vi "Get Grouped Channel Settings.vi"(9 "Type":T2(ring), 10 "Group Name":string, 11 "Group Settings":T3(array[cluster])) -> (1 "found?":bool, 2 "Channel Settings":T1(array[cluster]), 3 "Name based Group Settings":T3(array[cluster]))   [LabVIEW 2026, in "Template.lvlib" / "Template.lvclass"]
uses:
  Template.lvclass
  Template.lvclass/Template.ctl
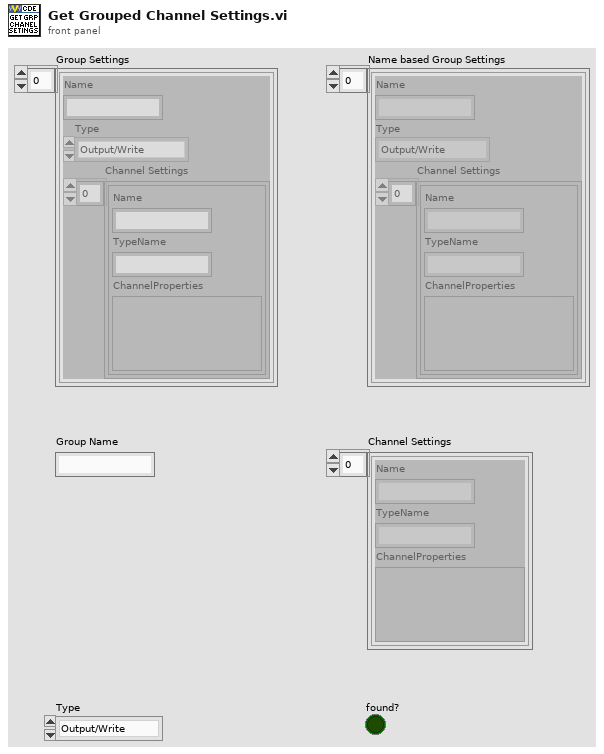
[diagram p1: front panel]
types:
  T1 = cluster{"Name":string, "TypeName":string, "ChannelProperties":variant}[]
  T2 = enum16{"Output/Write", "Input/Read", "Input/ReadWrite"}
  T3 = cluster{"Name":string, "Type":enum16{"Output/Write", "Input/Read", "Input/ReadWrite"}, "Channel Settings":cluster{"Name":string, "TypeName":string, "ChannelProperties":variant}[]}[]
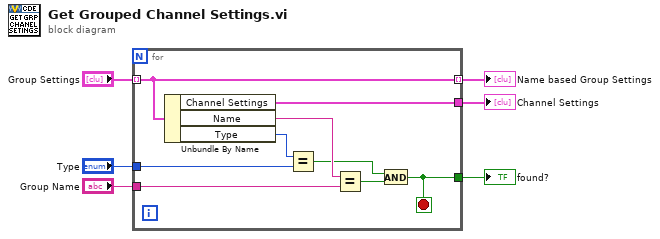
[diagram p0: block diagram]
diagram:
  n1 = for {
    tunnel: "Group Settings" -> [w8] mode=indexing
    tunnel: "Group Name" -> [w14]
    tunnel: [w11] -> w4
    tunnel: [w8] -> w3 mode=indexing
    tunnel: "Type" -> [w12]
    tunnel: [w7] -> w1
    stop <- w11 stop-if-true
    n2 = Unbundle By Name(w8) -> ("Channel Settings"=w7:T1, "Name"=w15:string, "Type"=w13:T2)
    n3 = Equal?(x=w13, y=w12) -> (x = y?=w9:bool)
    n4 = Equal?(x=w15, y=w14) -> (x = y?=w10:bool)
    n5 = And(x=w9, y=w10) -> (x .and. y?=w11:bool)
  }
  "found?" <- w4
  "Name based Group Settings" <- w3
  "Channel Settings" <- w1
